vi "Get Failure Action SEQ.vi"(8 "error in (no error)":errorcluster, 11 "Assert UID":string) -> (0 "error out":errorcluster, 1 "created new?":bool, 2 "Assert FA SEQ":refnum<queue>)   [LabVIEW 2016, in "Assert API Components.lvlib" / "Log Assert Core.lvlib"]
uses:
  Log Assert Core.lvlib
  Failure Actions.ctl
  Assert API Components.lvlib
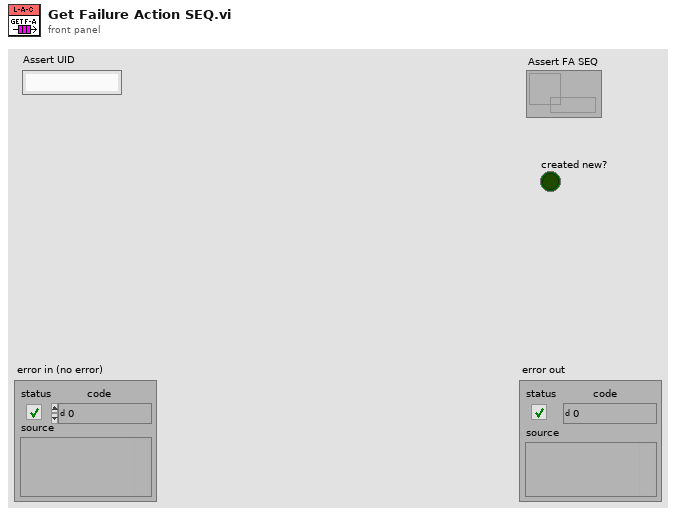
[diagram p1: front panel]
types:
  T1 = typedef "Assert API Components.lvlib/Failure Actions.ctl" = enum16{"None", "Log To File", "Pause Execution", "Abort Execution"}
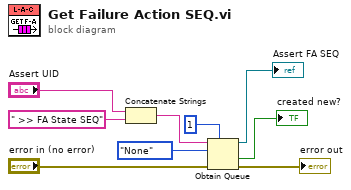
[diagram p0: block diagram]
diagram:
  n1 = Concatenate Strings("Assert UID", " >> FA State SEQ" ("string")) -> (w7:string)
  n2 = Obtain Queue(max queue size (-1, unlimited)=1, name (unnamed)=w7, element data type=Failure_Actions."None", error in (no error)="error in (no error)") -> (queue out=→"Assert FA SEQ":refnum<queue>, created new?=→"created new?":bool, error out=→"error out":errorcluster)  [unwired: 1 in]
